vi "Init Graph.vi"(8 "error in (no error)":errorcluster, 11 "Display Image in":refnum<class "Display Image.lvclass">) -> (0 "error out":errorcluster, 3 "Display Image out":refnum<class "Display Image.lvclass">)   [LabVIEW 2018, in "Display Image.lvclass"]
doc: "Este VI inicia o gráfico contido na classe com as dimensões do CCD em uso."
uses:
  Display Image.lvclass
  Display Image.lvclass/Display Image.ctl
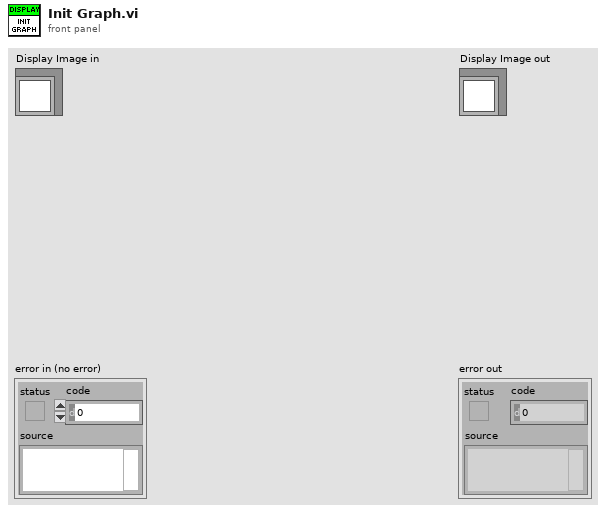
[diagram p1: front panel]
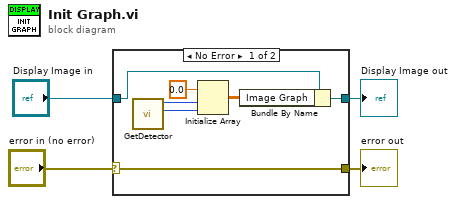
[diagram p0: block diagram]
diagram:
  n1 = case shown="No Error" "error in (no error)" {
    selector: "error in (no error)" -> [w11 w13]
    tunnel: [w11 w13] -> w3
    tunnel: [w6 w12] -> w1
    tunnel: "Display Image in" -> [w7 w12]
    frame No Error {
      n2 = call <userlib>:"GetDetector.vi"() -> ("ypixels"=w9:i32, "xpixels"=w10:i32)  [unwired: 4 in, 2 out]
      n3 = Initialize Array(0.0 ("element"), w10, w9) -> (w5:dbl[][])
      n4 = Bundle By Name(cluster=w7, "Image Graph"=w5) -> (w6:refnum<class "Display Image.lvclass">)
    }
    frame Error {
    }
  }
  "error out" <- w3
  "Display Image out" <- w1
